vi "get data definition.vi"(10 "channel classification":T1, 11 "Temperature Controller Logic runtime in":refnum<class "Temperature Controller Logic runtime.lvclass">) -> (1 "valid?":bool, 2 "index cluster":variant, 3 "Temperature Controller Logic runtime out":refnum<class "Temperature Controller Logic runtime.lvclass">)   [LabVIEW 2015, in "Temperature Controller Logic runtime.lvclass"]
uses:
  Temperature Controller Logic runtime.lvclass
  <vilib>/NI/Tag Bus Module Framework/channel/channel classification.ctl
  parameter user data.ctl
  result user data.ctl
  <vilib>/NI/Tag Bus Module Framework/channel/TBM channel.lvclass
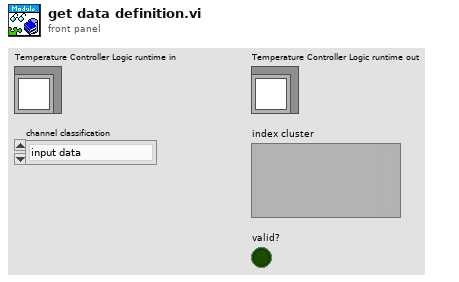
[diagram p1: front panel]
types:
  T1 = typedef "TBM channel.lvclass/channel classification.ctl" = enum16{"input data", "output data", "processing parameter", "processing result"}
  T2 = typedef "Temperature Controller Logic runtime.lvclass/parameter user data.ctl" = cluster{"Temperature":dbl, "setpoint":dbl, "output range high":dbl, "output range low":dbl, "Kc":dbl, "Ti":dbl, "Td":dbl, "Fan on?":bool}
  T3 = typedef "Temperature Controller Logic runtime.lvclass/result user data.ctl" = cluster{"fan":dbl, "lamp":dbl}
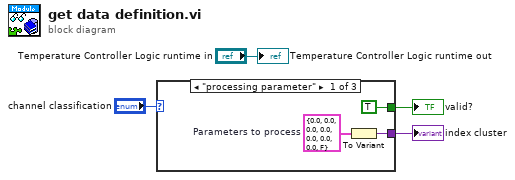
[diagram p0: block diagram]
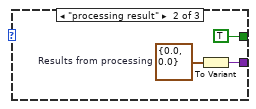
[diagram p2: hidden frame]
diagram:
  n1 = case shown="\"processing parameter\"" "channel classification" {
    tunnel: [TRUE TRUE _] -> w2
    tunnel: [w7 w10 _] -> w1
    frame "processing parameter" {
      w5 = T2 {"Temperature"=0.0, "setpoint"=0.0, "output range high"=0.0, "output range low"=0.0, "Kc"=0.0, "Ti"=0.0, "Td"=0.0, "Fan on?"=FALSE}  # Parameters to process
      n2 = To Variant(anything=w5) -> (Variant=w7:variant)
    }
    frame "processing result" {
      w8 = T3 {"fan"=0.0, "lamp"=0.0}  # Results from processing
      n3 = To Variant(anything=w8) -> (Variant=w10:variant)
    }
    frame Default {
    }
  }
  "valid?" <- w2
  "index cluster" <- w1
  "Temperature Controller Logic runtime out" <- "Temperature Controller Logic runtime in"
